vi "Ini key write (String).vi"(7 "Section":string, 8 "error in (no error)":errorcluster, 9 "Values (String)":string[](array[string]), 10 "Ini file interface":T2, 11 "Ini file refnum in":T1) -> (0 "error out":errorcluster, 3 "Ini file refnum out":T1)   [LabVIEW 2020]
uses:
  <vilib>/Utility/config.llb/Config Data RefNum.ctl
  Typedefs/Ini file interface (String).ctl
  <vilib>/Utility/config.llb/Write Key (String).vi
  <vilib>/Utility/config.llb/Read Key (String).vi
  <vilib>/Utility/config.llb/NI_LVConfig.lvlib
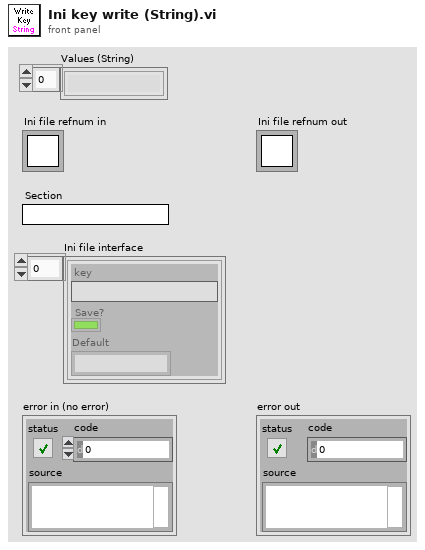
[diagram p1: front panel]
types:
  T1 = typedef "NI_LVConfig.lvlib/Config Data RefNum.ctl" = refnum<k1>
  T2 = typedef "Ini file interface (String).ctl" = cluster{"key":string, "Save?":bool, "Default":string}[]
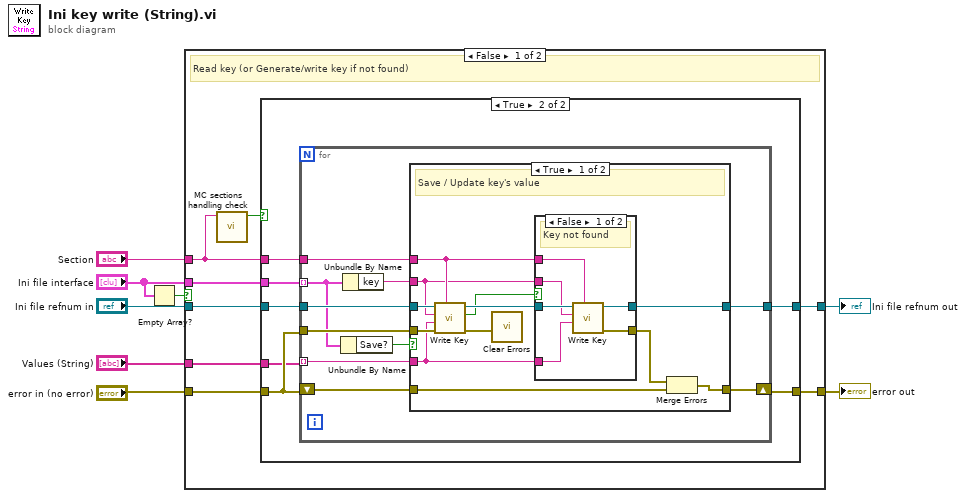
[diagram p0: block diagram]
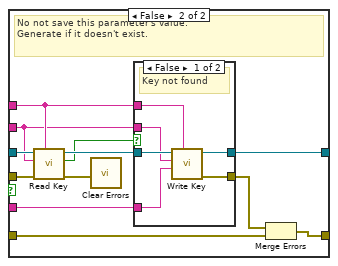
[diagram p4: hidden frame]
diagram:
  n1 = Empty Array?(array="Ini file interface") -> (empty?=w3:bool)
  n2 = case shown="False" w3 {
    tunnel: "Ini file refnum in" -> [w16 w75]
    tunnel: [w15 w75] -> w8
    tunnel: [w14 w74] -> w7
    tunnel: "error in (no error)" -> [w13 w74]
    tunnel: "Section" -> [w10 _]
    tunnel: "Ini file interface" -> [w12 _]
    tunnel: "Values (String)" -> [w11 _]
    frame False {
      # "Read key (or Generate/write key if not found)"
      n3 = call "MC sections handling check.vi"("Section name"=w10) -> ("Section is \"Initial MovCor Values\" AND MC is supported"=w9:bool)  [unwired: 10 in]
      n4 = case shown="True" w9 {
        tunnel: w16 -> [w18 w25]
        tunnel: [w18 w24] -> w15
        tunnel: [w17 w23] -> w14
        tunnel: w13 -> [w17 w22]
        tunnel: w10 -> [_ w21]
        tunnel: w12 -> [_ w20]
        tunnel: w11 -> [_ w19]
        frame False {
          # "The [Initial MovCor Values] section not handled when the MC UI is unavailable"
        }
        frame True {
          n5 = for {
            tunnel: w25 -> [w35]
            tunnel: w22 -> [w34]
            tunnel: [w33] -> w24
            shift-right: [w32] -> w23
            shift-left: w22 -> [w31]
            tunnel: w20 -> [w27] mode=indexing
            tunnel: w19 -> [w30] mode=indexing
            tunnel: w21 -> [w29]
            n6 = Unbundle By Name(w27) -> ("Save?"=w26:bool)
            n7 = Unbundle By Name(w27) -> ("key"=w28:string)
            n8 = case shown="True" w26 {
              tunnel: w35 -> [w47 w66]
              tunnel: w34 -> [w46 w65]
              tunnel: [w37 w56] -> w33
              tunnel: [w45 w64] -> w32
              tunnel: w31 -> [w44 w63]
              tunnel: w28 -> [w40 w59]
              tunnel: w30 -> [w38 w57]
              tunnel: w29 -> [w41 w60]
              frame True {
                # "Save / Update key's value"
                n9 = call-poly <vilib>:"Write Key.vi"("section"=w41, "error in (no error)"=w46, "value"=w38, "key"=w40, "refnum"=w47) -> ("error out"=w43:errorcluster, "found?"=w36:bool, "refnum out"=w42:T1)  [unwired: 4 in]
                n10 = call <vilib>:"Clear Errors.vi"("error in (no error)"=w43) -> ()  [unwired: 5 in, 2 out]
                n11 = case shown="False" w36 {
                  tunnel: w42 -> [w53 w54]
                  tunnel: [w52 w54] -> w37
                  tunnel: [w51 _] -> w39
                  tunnel: w41 -> [w50 _]
                  tunnel: w40 -> [w49 _]
                  tunnel: w38 -> [w48 _]
                  frame False {
                    # "Key not found"
                    n12 = call-poly <vilib>:"Write Key.vi"("section"=w50, "value"=w48, "key"=w49, "refnum"=w53) -> ("error out"=w51:errorcluster, "refnum out"=w52:T1)  [unwired: 5 in, 1 out]
                  }
                  frame True {
                    # "Key found"
                  }
                }
                n13 = Merge Errors(w39, w44) -> (w45:errorcluster)
              }
              frame False {
                # "No not save this parameter's value.\nGenerate if it doesn't exist."
                n14 = call-poly <vilib>:"Read Key.vi"("section"=w60, "error in (no error)"=w65, "key"=w59, "refnum"=w66) -> ("error out"=w62:errorcluster, "found?"=w55:bool, "refnum out"=w61:T1)  [unwired: 4 in, 1 out]
                n15 = call <vilib>:"Clear Errors.vi"("error in (no error)"=w62) -> ()  [unwired: 5 in, 2 out]
                n16 = case shown="False" w55 {
                  tunnel: w61 -> [w72 w73]
                  tunnel: [w71 w73] -> w56
                  tunnel: [w70 _] -> w58
                  tunnel: w60 -> [w69 _]
                  tunnel: w59 -> [w68 _]
                  tunnel: w57 -> [w67 _]
                  frame False {
                    # "Key not found"
                    n17 = call-poly <vilib>:"Write Key.vi"("section"=w69, "value"=w67, "key"=w68, "refnum"=w72) -> ("error out"=w70:errorcluster, "refnum out"=w71:T1)  [unwired: 5 in, 1 out]
                  }
                  frame True {
                    # "Key found"
                  }
                }
                n18 = Merge Errors(w58, w63) -> (w64:errorcluster)
              }
            }
          }
        }
      }
    }
    frame True {
      # "Setup array is empty"
    }
  }
  "Ini file refnum out" <- w8
  "error out" <- w7
